vi "target2.vi"() -> ()   [LabVIEW 2023]
panel:
  in  "y 2":dbl
  in  "x 3":dbl
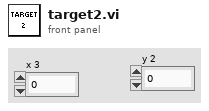
[diagram p1: front panel]
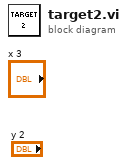
[diagram p0: block diagram]
diagram:
